vi "Automatic Teller Machine (ATM).vi"() -> ()   [LabVIEW 2018]
uses:
  controls/State.ctl
panel:
  in  "정지":bool
  in  "입력":bool
  in  "사용자 입력":string
  in  "오른쪽 버튼":T1
  out "오른쪽 메뉴":T2
  in  "왼쪽 버튼":T1
  out "왼쪽 메뉴":T2
  in  "카드 시뮬레이션":bool
  out "ATM 메시지":string
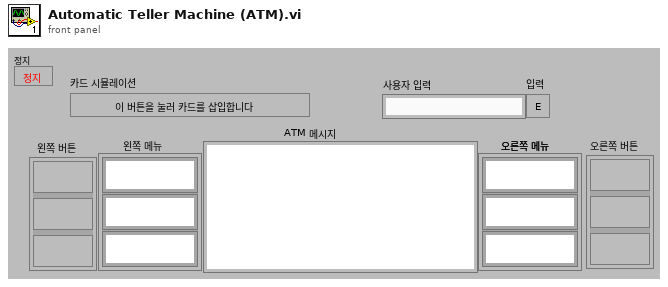
[diagram p1: front panel]
types:
  T1 = cluster{"함수 버튼":bool, "함수 버튼 2":bool, "함수 버튼 3":bool}
  T2 = cluster{"문자열":string, "문자열 2":string, "문자열 3":string}
  T3 = cluster{"오른쪽 메뉴":string, "문자열 2":string, "문자열 3":string}
  T4 = cluster{"왼쪽 메뉴":string, "문자열 2":string, "문자열 3":string}
  T5 = enum8{"Enabled", "Disabled", "Disabled and Grayed Out"}
  T6 = typedef "State.ctl" = enum16{"초기화", "시작", "ATM 카드 삽입", "계좌번호 입력 대기", "계좌번호 입력", "계좌 존재하지 않음", "계좌 존재", "노트", "입금", "입금 입력", "출금", "출금 입력", "잔고 충분", "잔고 불충분", "50불 즉시 지급", "사용하지 않음", "잔고 확인", "카드 반환 및 종료"}
  T7 = cluster{"왼쪽 메뉴":cluster{"왼쪽 메뉴":string, "문자열 2":string, "문자열 3":string}, "왼쪽 메뉴 2":cluster{"오른쪽 메뉴":string, "문자열 2":string, "문자열 3":string}, "왼쪽 버튼":cluster{"함수 버튼":bool, "왼쪽 버튼":bool, "함수 버튼 3":bool}, "왼쪽 버튼 2":cluster{"함수 버튼":bool, "오른쪽 버튼":bool, "함수 버튼 3":bool}, "입력 버튼":bool, "사용자 입력":string}
  T8 = cluster{"함수 버튼":bool, "왼쪽 버튼":bool, "함수 버튼 3":bool}
  T9 = cluster{"함수 버튼":bool, "오른쪽 버튼":bool, "함수 버튼 3":bool}
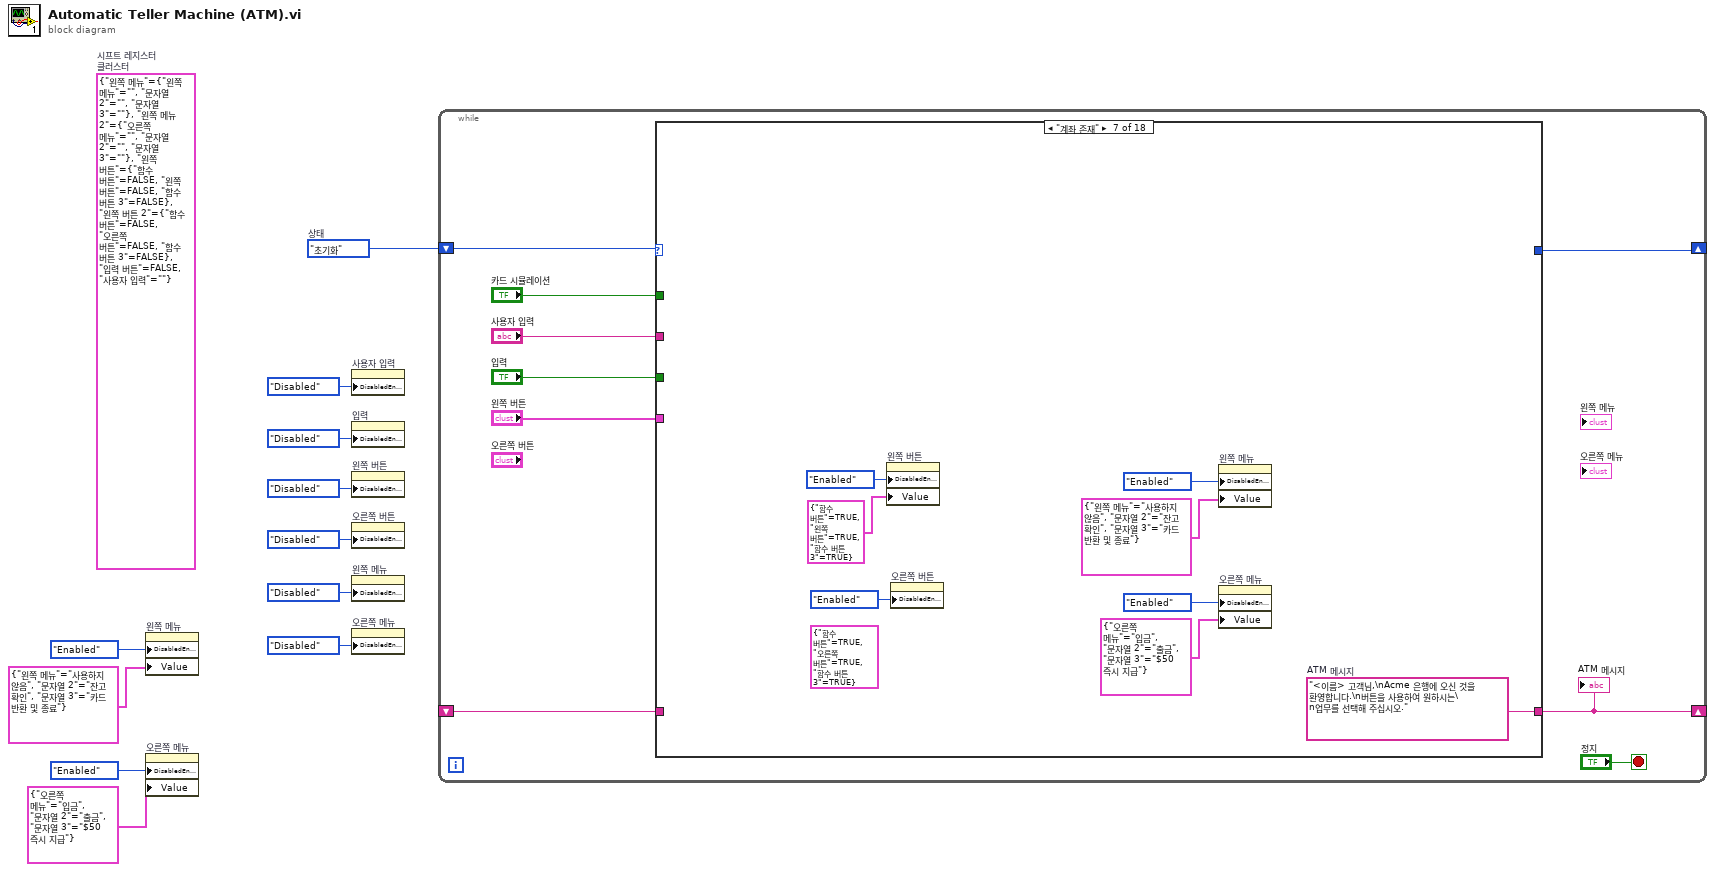
[diagram p0: block diagram]
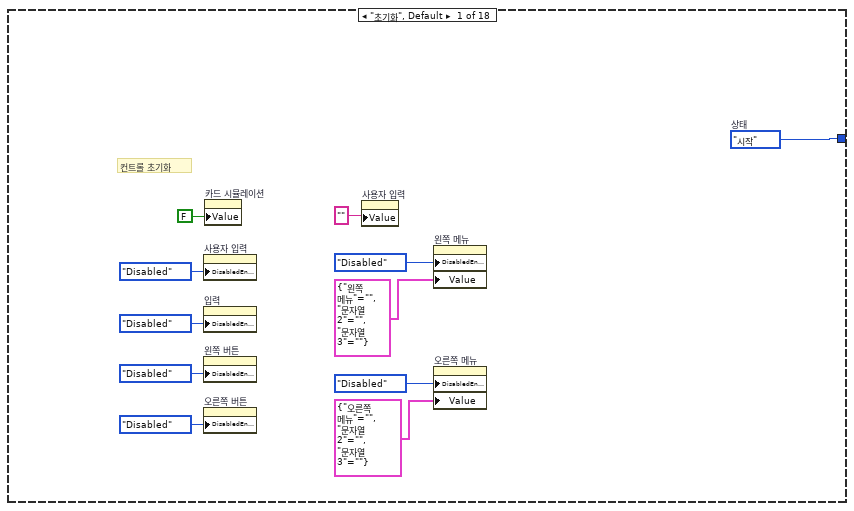
[diagram p2: hidden frame]
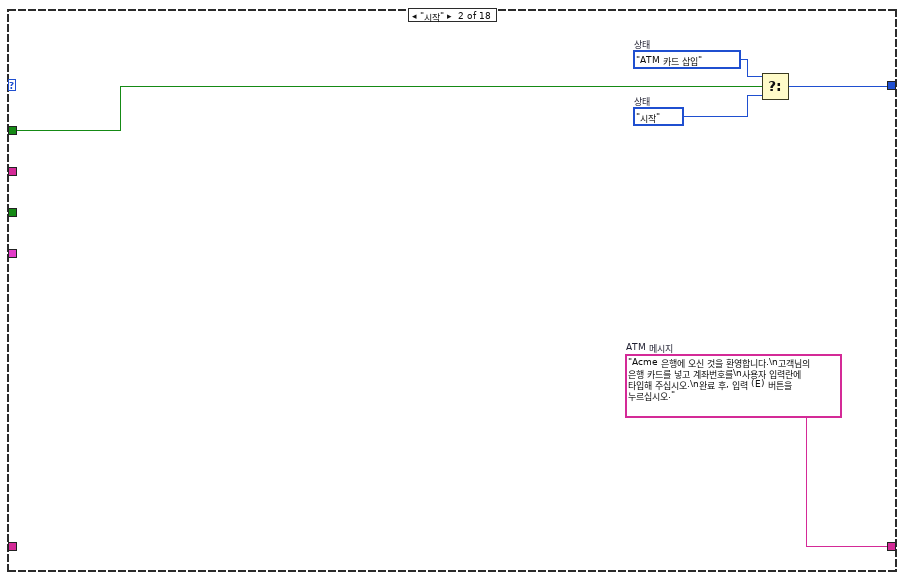
[diagram p3: hidden frame]
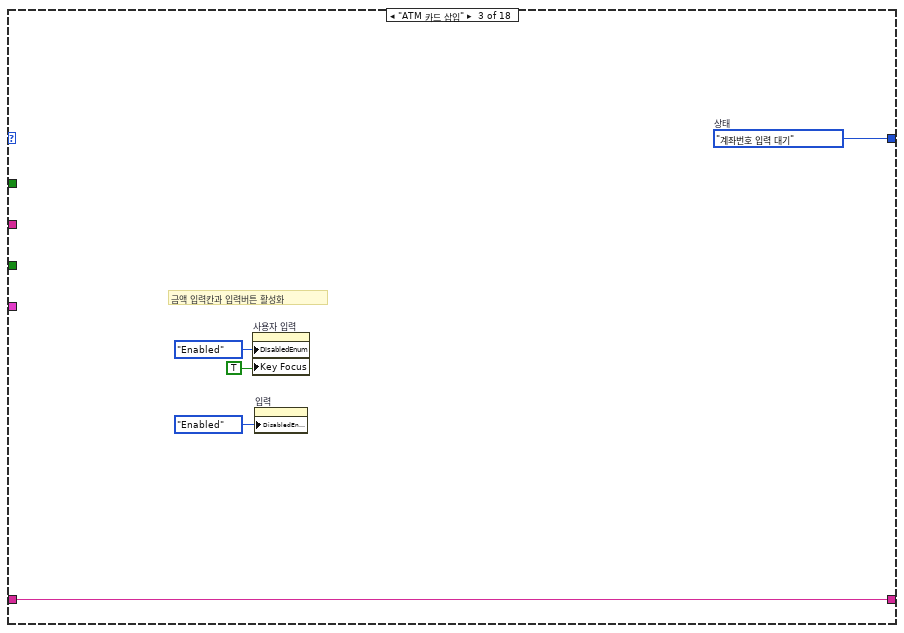
[diagram p4: hidden frame]
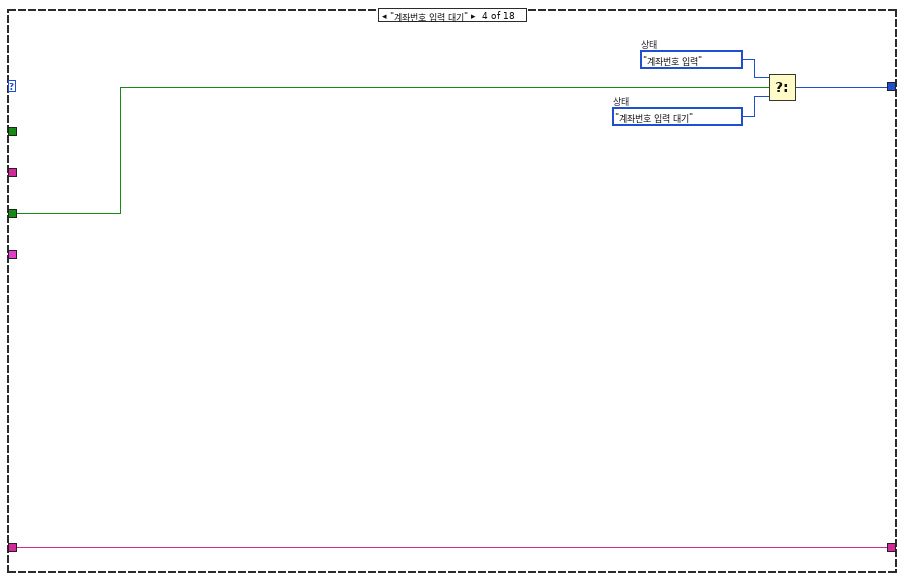
[diagram p5: hidden frame]
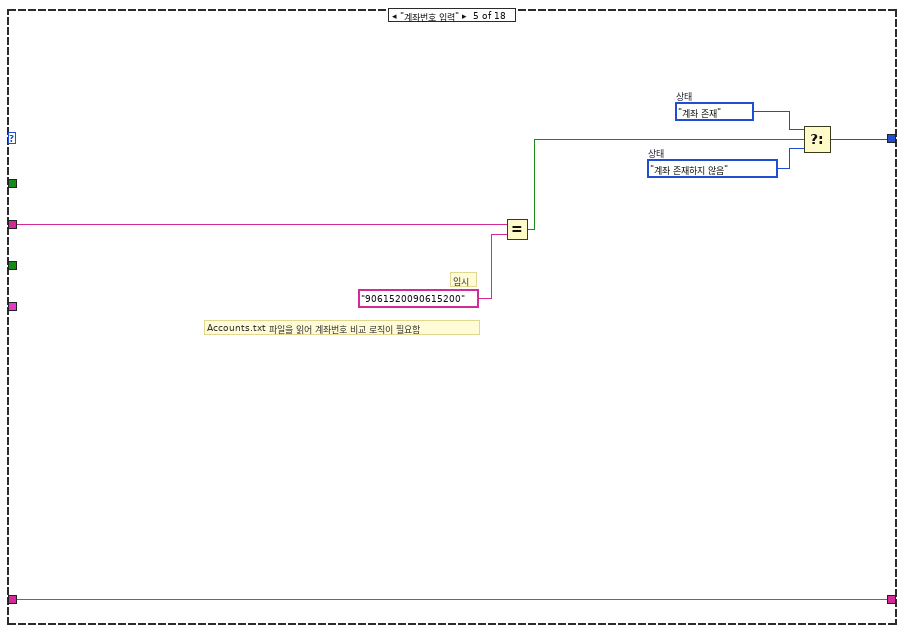
[diagram p6: hidden frame]
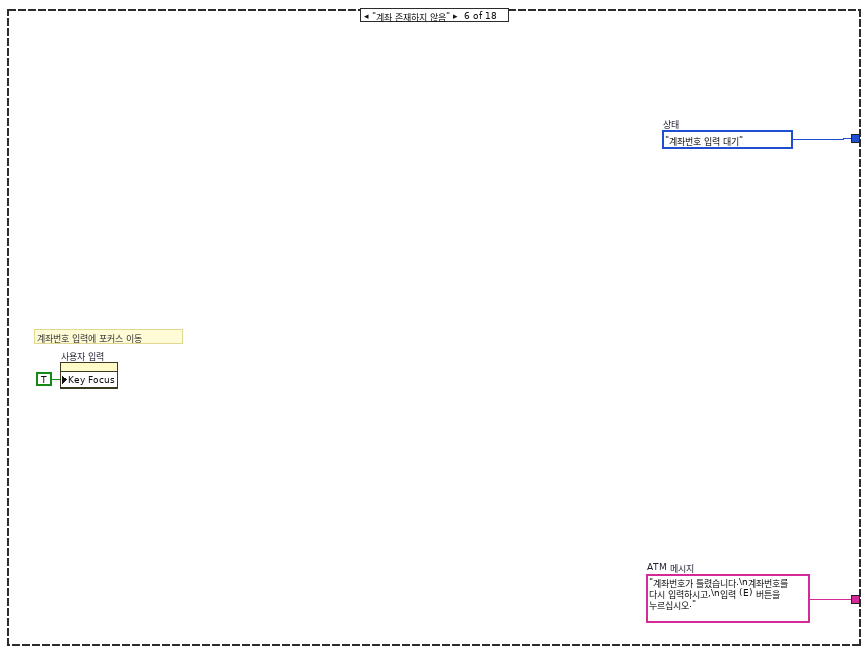
[diagram p7: hidden frame]
diagram:
  w11 = State."초기화"  # 상태
  (unwired) T7 {"왼쪽 메뉴"={"왼쪽 메뉴"="", "문자열 2"="", "문자열 3"=""}, "왼쪽 메뉴 2"={"오른쪽 메뉴"="", "문자열 2"="", "문자열 3"=""}, "왼쪽 버튼"={"함수 버튼"=FALSE, "왼쪽 버튼"=FALSE, "함수 버튼 3"=FALSE}, "왼쪽 버튼 2"={"함수 버튼"=FALSE, "오른쪽 버튼"=FALSE, "함수 버튼 3"=FALSE}, "입력 버튼"=FALSE, "사용자 입력"=""}  # 시프트 레지스터 클러스터
  n1 = property on="왼쪽 메뉴" class="Clust (엄격한)"("DisabledEnum"=T5."Enabled" ("비활성화"), "Value"=T4 {"왼쪽 메뉴"="사용하지 않음", "문자열 2"="잔고 확인", "문자열 3"="카드 반환 및 종료"} ("왼쪽 메뉴")) -> ()  [unwired: 2 in, 2 out]
  n2 = property on="오른쪽 메뉴" class="Clust (엄격한)"("DisabledEnum"=T5."Enabled" ("비활성화"), "Value"=T3 {"오른쪽 메뉴"="입금", "문자열 2"="출금", "문자열 3"="$50 즉시 지급"} ("왼쪽 메뉴 2")) -> ()  [unwired: 2 in, 2 out]
  n3 = property on="사용자 입력" class="Str"("DisabledEnum"=T5."Disabled" ("비활성화")) -> ()  [unwired: 2 in, 2 out]
  n4 = property on="입력" class="Bool"("DisabledEnum"=T5."Disabled" ("비활성화")) -> ()  [unwired: 2 in, 2 out]
  n5 = property on="왼쪽 버튼" class="Clust"("DisabledEnum"=T5."Disabled" ("비활성화")) -> ()  [unwired: 2 in, 2 out]
  n6 = property on="오른쪽 버튼" class="Clust"("DisabledEnum"=T5."Disabled" ("비활성화")) -> ()  [unwired: 2 in, 2 out]
  n7 = property on="왼쪽 메뉴" class="Clust (엄격한)"("DisabledEnum"=T5."Disabled" ("비활성화")) -> ()  [unwired: 2 in, 2 out]
  n8 = property on="오른쪽 메뉴" class="Clust (엄격한)"("DisabledEnum"=T5."Disabled" ("비활성화")) -> ()  [unwired: 2 in, 2 out]
  n9 = while {
    shift-right: [w19] -> _
    shift-left: w11 -> [w20]
    shift-right: [w13] -> _
    shift-left: _ -> [w12]
    stop <- "정지" stop-if-true
    n10 = case shown="\"계좌 존재\"" w20 {
      tunnel: [w31 w34 w38 w43 w49 w55 _ _ _ _ _ _ _ _ _ _ _ _] -> w19
      tunnel: "카드 시뮬레이션" -> [_ w35 _ _ _ _ _ _ _ _ _ _ _ _ _ _ _ _]
      tunnel: "입력" -> [_ _ _ w44 _ _ _ _ _ _ _ _ _ _ _ _ _ _]
      tunnel: "왼쪽 버튼" -> [_ _ _ _ _ _ _ _ _ _ _ _ _ _ _ _ _ _]
      tunnel: [_ w36 w37 w42 w47 w56 w60 _ _ _ _ _ _ _ _ _ _ _] -> w13
      tunnel: "사용자 입력" -> [_ _ _ _ w48 _ _ _ _ _ _ _ _ _ _ _ _ _]
      tunnel: w12 -> [_ _ w37 w42 w47 _ _ _ _ _ _ _ _ _ _ _ _ _]
      frame "초기화", Default {
        w31 = State."시작"  # 상태
        # "컨트롤 초기화"
        n11 = property on="사용자 입력" class="Str"("DisabledEnum"=T5."Disabled" ("비활성화")) -> ()  [unwired: 2 in, 2 out]
        n12 = property on="입력" class="Bool"("DisabledEnum"=T5."Disabled" ("비활성화")) -> ()  [unwired: 2 in, 2 out]
        n13 = property on="왼쪽 버튼" class="Clust"("DisabledEnum"=T5."Disabled" ("비활성화")) -> ()  [unwired: 2 in, 2 out]
        n14 = property on="오른쪽 버튼" class="Clust"("DisabledEnum"=T5."Disabled" ("비활성화")) -> ()  [unwired: 2 in, 2 out]
        n15 = property on="카드 시뮬레이션" class="Bool (엄격한)"("Value"=FALSE ("카드 시뮬레이션")) -> ()  [unwired: 2 in, 2 out]
        n16 = property on="사용자 입력" class="Str"("Value"="" ("사용자 입력")) -> ()  [unwired: 2 in, 2 out]
        n17 = property on="왼쪽 메뉴" class="Clust (엄격한)"("DisabledEnum"=T5."Disabled" ("비활성화"), "Value"=T4 {"왼쪽 메뉴"="", "문자열 2"="", "문자열 3"=""} ("왼쪽 메뉴")) -> ()  [unwired: 2 in, 2 out]
        n18 = property on="오른쪽 메뉴" class="Clust (엄격한)"("DisabledEnum"=T5."Disabled" ("비활성화"), "Value"=T3 {"오른쪽 메뉴"="", "문자열 2"="", "문자열 3"=""} ("왼쪽 메뉴 2")) -> ()  [unwired: 2 in, 2 out]
      }
      frame "시작" {
        w32 = State."시작"  # 상태
        w33 = State."ATM 카드 삽입"  # 상태
        w36 = "Acme 은행에 오신 것을 환영합니다.\n고객님의 은행 카드를 넣고 계좌번호를\n사용자 입력란에 타입해 주십시오.\n완료 후, 입력 (E) 버튼을 누르십시오."  # ATM 메시지
        n19 = Select(t=w33, s=w35, f=w32) -> (s? t:f=w34:T6)
      }
      frame "ATM 카드 삽입" {
        w38 = State."계좌번호 입력 대기"  # 상태
        # "금액 입력칸과 입력버튼 활성화"
        n20 = property on="사용자 입력" class="Str"("DisabledEnum"=T5."Enabled" ("비활성화"), "Key Focus"=TRUE ("키 포커스")) -> ()  [unwired: 2 in, 2 out]
        n21 = property on="입력" class="Bool"("DisabledEnum"=T5."Enabled" ("비활성화")) -> ()  [unwired: 2 in, 2 out]
      }
      frame "계좌번호 입력 대기" {
        w45 = State."계좌번호 입력 대기"  # 상태
        w46 = State."계좌번호 입력"  # 상태
        n22 = Select(t=w46, s=w44, f=w45) -> (s? t:f=w43:T6)
      }
      frame "계좌번호 입력" {
        w52 = State."계좌 존재하지 않음"  # 상태
        w53 = State."계좌 존재"  # 상태
        # "Accounts.txt 파일을 읽어 계좌번호 비교 로직이 필요함"
        # "임시"
        n23 = Equal?(x=w48, y="9061520090615200") -> (x = y?=w51:bool)
        n24 = Select(t=w53, s=w51, f=w52) -> (s? t:f=w49:T6)
      }
      frame "계좌 존재하지 않음" {
        w55 = State."계좌번호 입력 대기"  # 상태
        w56 = "계좌번호가 틀렸습니다.\n계좌번호를 다시 입력하시고,\n입력 (E) 버튼을 누르십시오."  # ATM 메시지
        # "계좌번호 입력에 포커스 이동"
        n25 = property on="사용자 입력" class="Str"("Key Focus"=TRUE ("키 포커스")) -> ()  [unwired: 2 in, 2 out]
      }
      frame "계좌 존재" {
        (unwired) T9 {"함수 버튼"=TRUE, "오른쪽 버튼"=TRUE, "함수 버튼 3"=TRUE} ("왼쪽 버튼 2")
        w60 = "<이름> 고객님,\nAcme 은행에 오신 것을 환영합니다.\n버튼을 사용하여 원하시는\n업무를 선택해 주십시오."  # ATM 메시지
        n26 = property on="왼쪽 버튼" class="Clust"("DisabledEnum"=T5."Enabled" ("비활성화"), "Value"=T8 {"함수 버튼"=TRUE, "왼쪽 버튼"=TRUE, "함수 버튼 3"=TRUE} ("왼쪽 버튼")) -> ()  [unwired: 2 in, 2 out]
        n27 = property on="오른쪽 버튼" class="Clust"("DisabledEnum"=T5."Enabled" ("비활성화")) -> ()  [unwired: 2 in, 2 out]
        n28 = property on="왼쪽 메뉴" class="Clust (엄격한)"("DisabledEnum"=T5."Enabled" ("비활성화"), "Value"=T4 {"왼쪽 메뉴"="사용하지 않음", "문자열 2"="잔고 확인", "문자열 3"="카드 반환 및 종료"} ("왼쪽 메뉴")) -> ()  [unwired: 2 in, 2 out]
        n29 = property on="오른쪽 메뉴" class="Clust (엄격한)"("DisabledEnum"=T5."Enabled" ("비활성화"), "Value"=T3 {"오른쪽 메뉴"="입금", "문자열 2"="출금", "문자열 3"="$50 즉시 지급"} ("왼쪽 메뉴 2")) -> ()  [unwired: 2 in, 2 out]
      }
      frame "노트" {
      }
      frame "입금" {
      }
      frame "입금 입력" {
      }
      frame "출금" {
      }
      frame "출금 입력" {
      }
      frame "잔고 충분" {
      }
      frame "잔고 불충분" {
      }
      frame "50불 즉시 지급" {
      }
      frame "사용하지 않음" {
      }
      frame "잔고 확인" {
      }
      frame "카드 반환 및 종료" {
      }
    }
    "ATM 메시지" <- w13
  }
